vi "EUI_3.vi"() -> ()   [LabVIEW 2018]
uses:
  <vilib>/FPGAPlugInAG/cRIO-9034/niLvFpga_Open_cRIO-9034.vi
  <vilib>/rvi/interface/common/dynamic/niFpgaDynamicAddResources.vi
  <vilib>/FPGAPlugInAG/Dynamic/niLvFpga_Run_Dynamic.vi
  <vilib>/Utility/error.llb/Error Cluster From Error Code.vi
  <vilib>/rvi/errors/niLvFpgaAdjustHostInterfaceError.vi
  <vilib>/rvi/interface/nirviOpenFPGA/nirviOpenFPGA.xnode
  Bitfiles/NiFpga_VMS_3_Controller.lvbitx
  VMS_3_Controller.vi
  <vilib>/rvi/interface/nirviMethod/nirviMethod.xnode
  <vilib>/rvi/interface/nirviReadWriteControl/nirviReadWriteControl.xnode
  <vilib>/rvi/interface/Simulation/niFpgaSimulationCallBeginRW.vi
  NiFpgaLv.dll
  <vilib>/FPGAPlugInAG/Dynamic/niLvFpga_ReadFifo_Dynamic.vi
  <vilib>/rvi/errors/niLvFpgaMergeErrorWithErrorCode.vi
panel:
  out "FIFO full":bool
  out "last readout error":errorcluster
  in  "Period (ms)":i32=5
  out "error out":errorcluster
  out "Stopped":bool
  in  "Output type":T1(ring)
  out "Timeouted":bool
  out "Ticks":u64
  out "Ready":bool
  out "Accelerometers":sgl[](graph)
  in  "Operate":bool
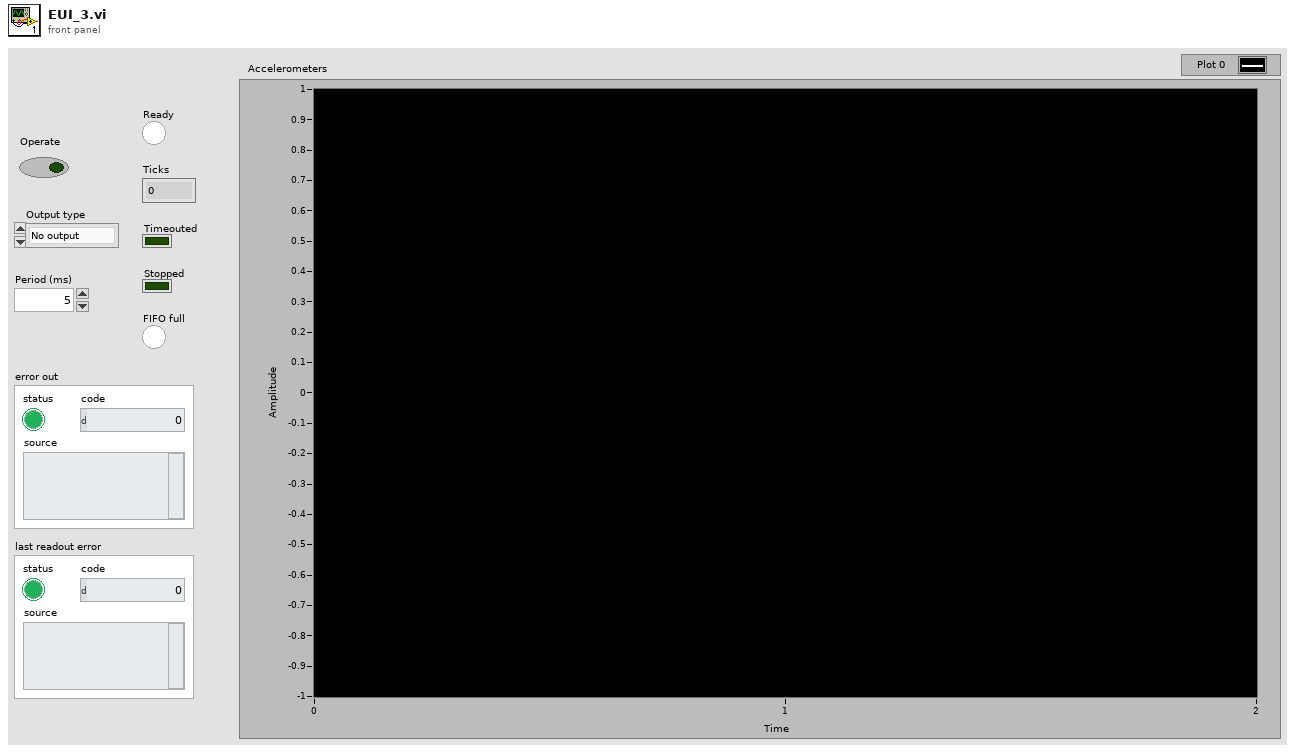
[diagram p1: front panel]
types:
  T1 = enum16{"No output", "Minimum", "Maximum", "Average"}
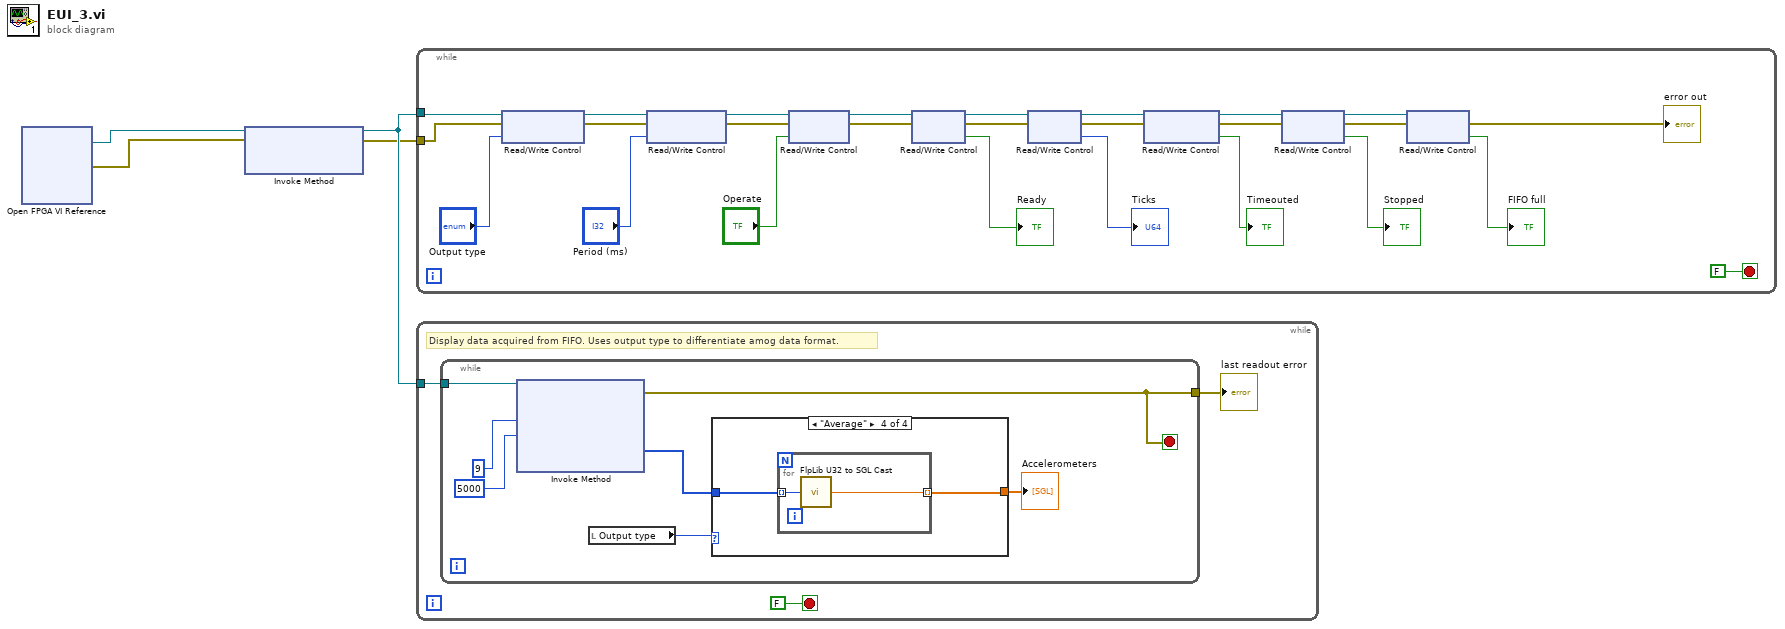
[diagram p0: block diagram]
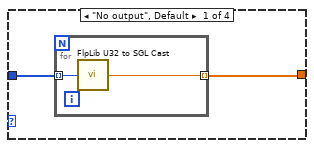
[diagram p2: hidden frame]
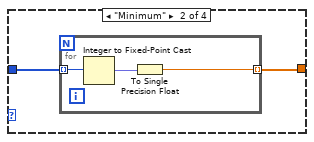
[diagram p3: hidden frame]
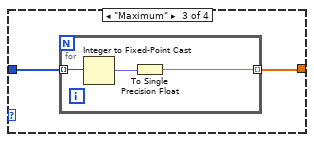
[diagram p4: hidden frame]
diagram:
  n1 = xnode "Open FPGA VI Reference"() -> ("FPGA VI Reference Out"=w1:refnum<k20>, "error out"=w2:errorcluster)  [unwired: 2 in]
  n2 = xnode "Invoke Method"("FPGA VI Reference In"=w1, "error in"=w2) -> ("FPGA VI Reference Out"=w4:refnum<k20>, "error out"=w3:errorcluster)  [unwired: 1 in]
  n3 = while {
    tunnel: w4 -> [w29]
    tunnel: w3 -> [w17]
    stop <- FALSE stop-if-true
    n4 = xnode "Read/Write Control"("FPGA VI Reference In"=w29, "error in"=w17, "Output type"="Output type") -> ("FPGA VI Reference Out"=w21:refnum<k20>, "error out"=w11:errorcluster)
    n5 = xnode "Read/Write Control"("FPGA VI Reference In"=w21, "error in"=w11, "Period (ms)"="Period (ms)") -> ("FPGA VI Reference Out"=w12:refnum<k20>, "error out"=w10:errorcluster)
    n6 = xnode "Read/Write Control"("FPGA VI Reference In"=w12, "error in"=w10, "Operate"="Operate") -> ("FPGA VI Reference Out"=w27:refnum<k20>, "error out"=w16:errorcluster)
    n7 = xnode "Read/Write Control"("FPGA VI Reference In"=w27, "error in"=w16) -> ("FPGA VI Reference Out"=w25:refnum<k20>, "error out"=w15:errorcluster, "Ready"=→"Ready":bool)
    n8 = xnode "Read/Write Control"("FPGA VI Reference In"=w25, "error in"=w15) -> ("FPGA VI Reference Out"=w23:refnum<k20>, "error out"=w14:errorcluster, "Ticks"=→"Ticks":u64)
    n9 = xnode "Read/Write Control"("FPGA VI Reference In"=w23, "error in"=w14) -> ("FPGA VI Reference Out"=w19:refnum<k20>, "error out"=w13:errorcluster, "Timeouted"=→"Timeouted":bool)
    n10 = xnode "Read/Write Control"("FPGA VI Reference In"=w19, "error in"=w13) -> ("FPGA VI Reference Out"=w6:refnum<k20>, "error out"=w8:errorcluster, "Stopped"=→"Stopped":bool)
    n11 = xnode "Read/Write Control"("FPGA VI Reference In"=w6, "error in"=w8) -> ("error out"=→"error out":errorcluster, "FIFO full"=→"FIFO full":bool)  [unwired: 1 out]
  }
  n12 = while {
    tunnel: w4 -> [w33]
    stop <- FALSE stop-if-true
    # "Display data acquired from FIFO. Uses output type to differentiate amog data format."
    n13 = while {
      tunnel: w33 -> [w40]
      tunnel: [w36] -> w31
      stop <- w36 stop-if-true
      n14 = xnode "Invoke Method"("FPGA VI Reference In"=w40, "Number of Elements"=u32 9, "Timeout (ms)"=5000) -> ("error out"=w36:errorcluster, "Data"=w38:u32[])  [unwired: 1 in, 2 out]
      n15 = local read "Output type"() -> (w34:T1)
      n16 = case shown="\"Average\"" w34 {
        tunnel: w38 -> [w42 w46 w51 w56]
        tunnel: [w41 w45 w50 w55] -> w35
        frame "No output", Default {
          n17 = for {
            tunnel: w42 -> [w44] mode=indexing
            tunnel: [w43] -> w41 mode=indexing
            n18 = call <userlib>:"FlpLib U32 to SGL Cast.vi"("x"=w44) -> ("y"=w43:sgl)  [unwired: 4 in]
          }
        }
        frame "Minimum" {
          n19 = for {
            tunnel: w46 -> [w49] mode=indexing
            tunnel: [w47] -> w45 mode=indexing
            n20 = Integer to Fixed-Point Cast(integer=w49) -> (fixed-point=w48:fxp<+/-,24,4>)  [unwired: 1 in]
            n21 = To Single Precision Float(number=w48) -> (single precision float=w47:sgl)
          }
        }
        frame "Maximum" {
          n22 = for {
            tunnel: w51 -> [w54] mode=indexing
            tunnel: [w52] -> w50 mode=indexing
            n23 = Integer to Fixed-Point Cast(integer=w54) -> (fixed-point=w53:fxp<+/-,24,4>)  [unwired: 1 in]
            n24 = To Single Precision Float(number=w53) -> (single precision float=w52:sgl)
          }
        }
        frame "Average" {
          n25 = for {
            tunnel: w56 -> [w58] mode=indexing
            tunnel: [w57] -> w55 mode=indexing
            n26 = call <userlib>:"FlpLib U32 to SGL Cast.vi"("x"=w58) -> ("y"=w57:sgl)  [unwired: 4 in]
          }
        }
      }
      "Accelerometers" <- w35
    }
    "last readout error" <- w31
  }
